vi "Get Skeletal Frame.vi"(8 "error in (no error)":errorcluster, 11 "Kinect Session in":refnum<class "Kinect Session.lvclass">) -> (0 "error out":errorcluster, 2 "Skeletal Data":T1(array[cluster]), 3 "Kinect Session out":refnum<class "Kinect Session.lvclass">)   [LabVIEW 2011, in "Kinect Library.lvlib"]
doc: "THIS FUNCTION DOES NOT FUNCTION YET.\n\nIt will eventually create a cluster for the user of the post-processed Skeletal information."
uses:
  Kinect Library.lvlib
  Kinect Session Class/Kinect Session.lvclass
  Microsoft.Kinect
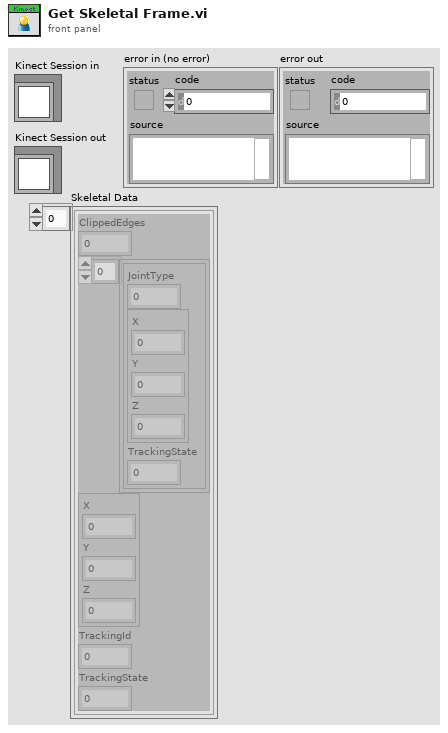
[diagram p1: front panel]
types:
  T1 = cluster{"ClippedEdges":i32, cluster{"JointType":i32, cluster{"X":sgl, "Y":sgl, "Z":sgl}, "TrackingState":i32}[], cluster{"X":sgl, "Y":sgl, "Z":sgl}, "TrackingId":i32, "TrackingState":i32}[]
  T2 = cluster{"JointType":i32, cluster{"X":sgl, "Y":sgl, "Z":sgl}, "TrackingState":i32}
  T3 = cluster{"ClippedEdges":i32, cluster{"JointType":i32, cluster{"X":sgl, "Y":sgl, "Z":sgl}, "TrackingState":i32}[], cluster{"X":sgl, "Y":sgl, "Z":sgl}, "TrackingId":i32, "TrackingState":i32}
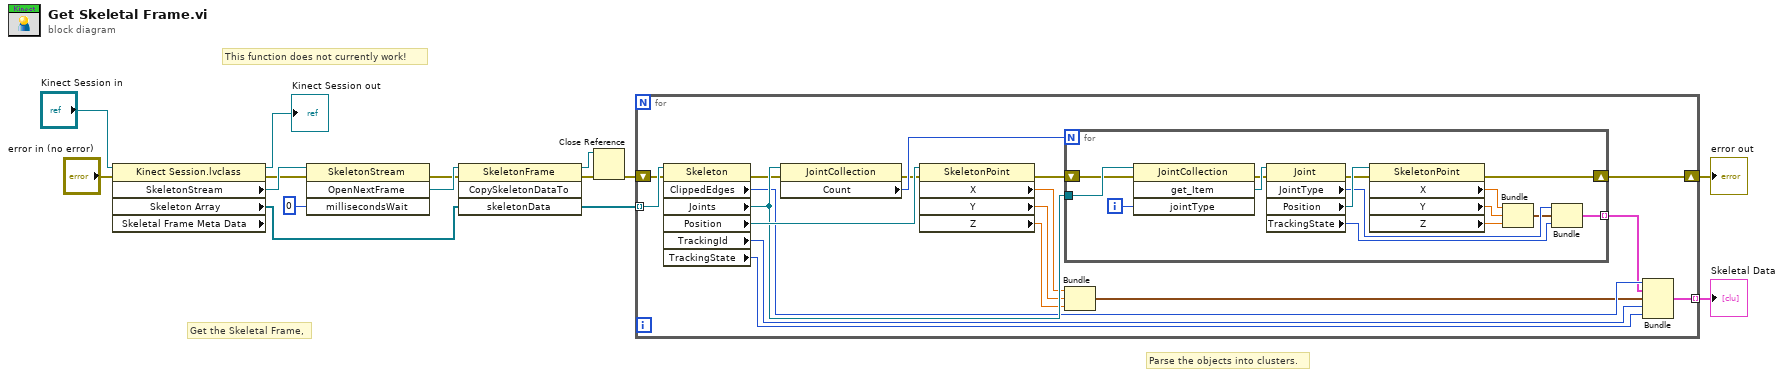
[diagram p0: block diagram]
diagram:
  # "Parse the objects into clusters."
  # "Get the Skeletal Frame,"
  # "This function does not currently work!"
  n1 = property class="Kinect Session.lvclass" props=["SkeletonStream", "Skeleton Array", "Skeletal Frame Meta Data"](reference="Kinect Session in", error in="error in (no error)") -> (reference out=→"Kinect Session out":refnum<class "Kinect Session.lvclass">, error out=w4:errorcluster, "SkeletonStream"=w7:refnum<k24>, "Skeleton Array"=w8:refnum<k24>[])  [unwired: 1 out]
  n2 = invoke class="SkeletonStream" method="OpenNextFrame"(reference=w7, error in=w4, "millisecondsWait"=0) -> (error out=w11:errorcluster, "OpenNextFrame"=w13:refnum<k24>)  [unwired: 1 in, 2 out]
  n3 = invoke class="SkeletonFrame" method="CopySkeletonDataTo"(reference=w13, error in=w11, "skeletonData"=w8) -> (reference out=w14:refnum<k24>, error out=w12:errorcluster, "skeletonData"=w15:refnum<k24>[])  [unwired: 1 in, 1 out]
  n4 = Close Reference(reference=w14, error in (no error)=w12) -> (error out=w10:errorcluster)
  n5 = for {
    tunnel: w15 -> [w33] mode=indexing
    tunnel: [w21] -> w9 mode=indexing
    shift-right: [w16] -> w3
    shift-left: w10 -> [w17]
    n6 = property class="Skeleton"(reference=w33, error in=w17) -> (error out=w20:errorcluster, "ClippedEdges"=w26:i32, "Joints"=w31:refnum<k24>, "Position"=w32:refnum<k24>, "TrackingId"=w23:i32, "TrackingState"=w22:i32)  [unwired: 1 out]
    n7 = property class="JointCollection"(reference=w31, error in=w20) -> (error out=w19:errorcluster, "Count"=w30:i32)  [unwired: 1 out]
    n8 = property class="SkeletonPoint"(reference=w32, error in=w19) -> (error out=w18:errorcluster, "X"=w29:sgl, "Y"=w28:sgl, "Z"=w27:sgl)  [unwired: 1 out]
    n9 = for {
      N: w30 -> [_]
      tunnel: w31 -> [w48]
      tunnel: [w38] -> w25 mode=indexing
      shift-right: [w34] -> w16
      shift-left: w18 -> [w37]
      i -> [w47]
      n10 = invoke class="JointCollection" method="get_Item"(reference=w48, error in=w37, "jointType"=w47) -> (error out=w36:errorcluster, "get_Item"=w46:refnum<k24>)  [unwired: 1 in, 2 out]
      n11 = property class="Joint"(reference=w46, error in=w36) -> (error out=w35:errorcluster, "JointType"=w41:i32, "Position"=w45:refnum<k24>, "TrackingState"=w39:i32)  [unwired: 1 out]
      n12 = property class="SkeletonPoint"(reference=w45, error in=w35) -> (error out=w34:errorcluster, "X"=w44:sgl, "Y"=w43:sgl, "Z"=w42:sgl)  [unwired: 1 out]
      n13 = Bundle("X"=w44, "Y"=w43, "Z"=w42) -> (w40:cluster{"X":sgl, "Y":sgl, "Z":sgl})  [unwired: 1 in]
      n14 = Bundle("JointType"=w41, w40, "TrackingState"=w39) -> (w38:T2)  [unwired: 1 in]
    }
    n15 = Bundle("X"=w29, "Y"=w28, "Z"=w27) -> (w24:cluster{"X":sgl, "Y":sgl, "Z":sgl})  [unwired: 1 in]
    n16 = Bundle("ClippedEdges"=w26, w25, w24, "TrackingId"=w23, "TrackingState"=w22) -> (w21:T3)  [unwired: 1 in]
  }
  "Skeletal Data" <- w9
  "error out" <- w3
